vi "Check_Execution_Row.vi"(0 "Execution Row":T1 {"Row Duration (mins)" format="%#.1f"; "Row No" min=0; "Trace Gas Concentration (%)" min=0.0 format="%#.2f"; "Emission Rate (l/min)" format="%#.2f"; "Tunnel Speed" format="%#.2f"; "Start X" format="%#.2f"; "Start Y" format="%#.2f"; "Start Z" format="%#.2f"; "End X" format="%#.2f"; "End Y" format="%#.2f"; "End Z" format="%#.2f"; "Averaging time (min)" min=0.0 format="%#.2f"}, 3 "Synchronization Start No":i32=1 min=1 max=100, 4 "Row Index":i32, 5 "Max Tunnel Speed":dbl format="%.2f") -> (6 "Editted Row":bool, 7 "Execution Row Out":T1 {"Row Duration (mins)" format="%#.1f"; "Row No" min=0; "Trace Gas Concentration (%)" min=0.0 format="%#.2f"; "Emission Rate (l/min)" format="%#.2f"; "Tunnel Speed" format="%#.2f"; "Start X" format="%#.2f"; "Start Y" format="%#.2f"; "Start Z" format="%#.2f"; "End X" format="%#.2f"; "End Y" format="%#.2f"; "End Z" format="%#.2f"; "Averaging time (min)" min=0.0 format="%#.2f"}, 9 "Continue?":bool, 10 "Error Comments":string)   [LabVIEW 2013]
uses:
  Traverse_cluster.ctl
  Spacing.ctl
  Controls/Multi_run_mode.ctl
  Controls/User_Specific_mode.ctl
  Controls/Tunnel_Coordinates.ctl
  ADAM Client/Sub VIs/ADAM Controls/Channel_names.ctl
  Globals/Extra_Commands_Global.vi
  Globals/Constants_global.vi
  Globals/Trav_pos_global.vi
panel:
  out "Traverse line Out":T1 {"Row Duration (mins)" format="%#.1f"; "Row No" min=0; "Trace Gas Concentration (%)" min=0.0 format="%#.2f"; "Emission Rate (l/min)" format="%#.2f"; "Tunnel Speed" format="%#.2f"; "Start X" format="%#.2f"; "Start Y" format="%#.2f"; "Start Z" format="%#.2f"; "End X" format="%#.2f"; "End Y" format="%#.2f"; "End Z" format="%#.2f"; "Averaging time (min)" min=0.0 format="%#.2f"}
  out "Fixed Axis":bool[](array[boolean])
  out "Filenames":string[](array[string])
  out "Current Sync Number":i32
  out "Checks":string[](array[string])
  in  "Edit in Excel":bool
  in  "OK":bool
  # "X           Y            Z"
  # "Start"
  # "End"
  # "X           Y            Z"
  # "Start"
  # "End"
  # "X           Y            Z"
  # "Start"
  # "End"
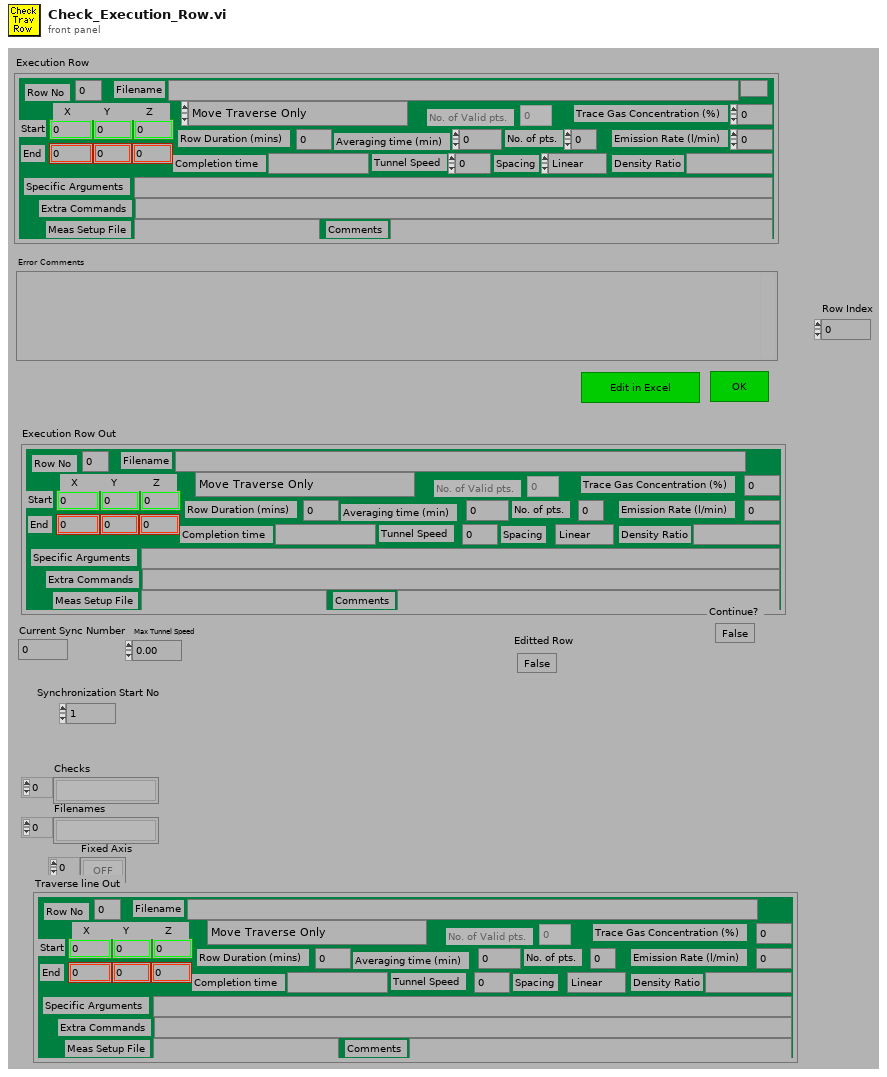
[diagram p1: front panel]
types:
  T1 = typedef "Traverse_cluster.ctl" = cluster{"Start X":dbl, "Start Y":dbl, "Start Z":dbl, "End X":dbl, "End Y":dbl, "End Z":dbl, "No. of pts.":i32, "Spacing":T2, "Filename":path, "Tunnel Speed":dbl, "Averaging time (min)":dbl, "Extra Commands":string, "Specific Arguments":string, "Emission Rate (l/min)":dbl, "Trace Gas Concentration (%)":dbl, "Density Ratio":string, "Comments":string, "Row No":i32, "Row Type Selector":T3, "Completion time":string, "Row Duration (mins)":dbl, "No. of Valid pts.":i32, "Meas Setup File":string}
  T2 = typedef "Spacing.ctl" = enum16{"Linear", "Log", "Gauss", "Specified", "N/A"}
  T3 = typedef "Multi_run_mode.ctl" = enum16{"Move Traverse Only", "Set Tunnel Speed Only", "Set Source Only", "Set Measurement Conditions", "Single Measurement", "Vertical Profile", "Lateral Profile", "Longitudinal Profile", "Explore Volume", "Multi-Axis Profile", "Auto Calibrate", "Meas Fast FID Bkgnd", "Check Beam Power", "Scanning Valve Measurement", "Run VI Named:", "Set ADAM Ch", "Wait (minutes)", "Send Message", "Synchronize With:", "Fall Back to this Row", "Turn Off Row Repeating", "Blank Row", "Traverse 3D Volume"}
  T4 = enum16{"All Channel Names", "Valid Channel Names"}
  T5 = typedef "User_Specific_mode.ctl" = enum16{"Check VI only", "Run VI"}
  T6 = typedef "Tunnel_Coordinates.ctl" = enum16{"Work in Tunnel Coordinates", "Work in Model Coordinates"}
  T7 = enum16{"Zero or one", "One", "Zero or more", "One or more"}
  T8 = typedef "Channel_names.ctl" = enum16{"Active Only", "Active + Off", "All Channels"}
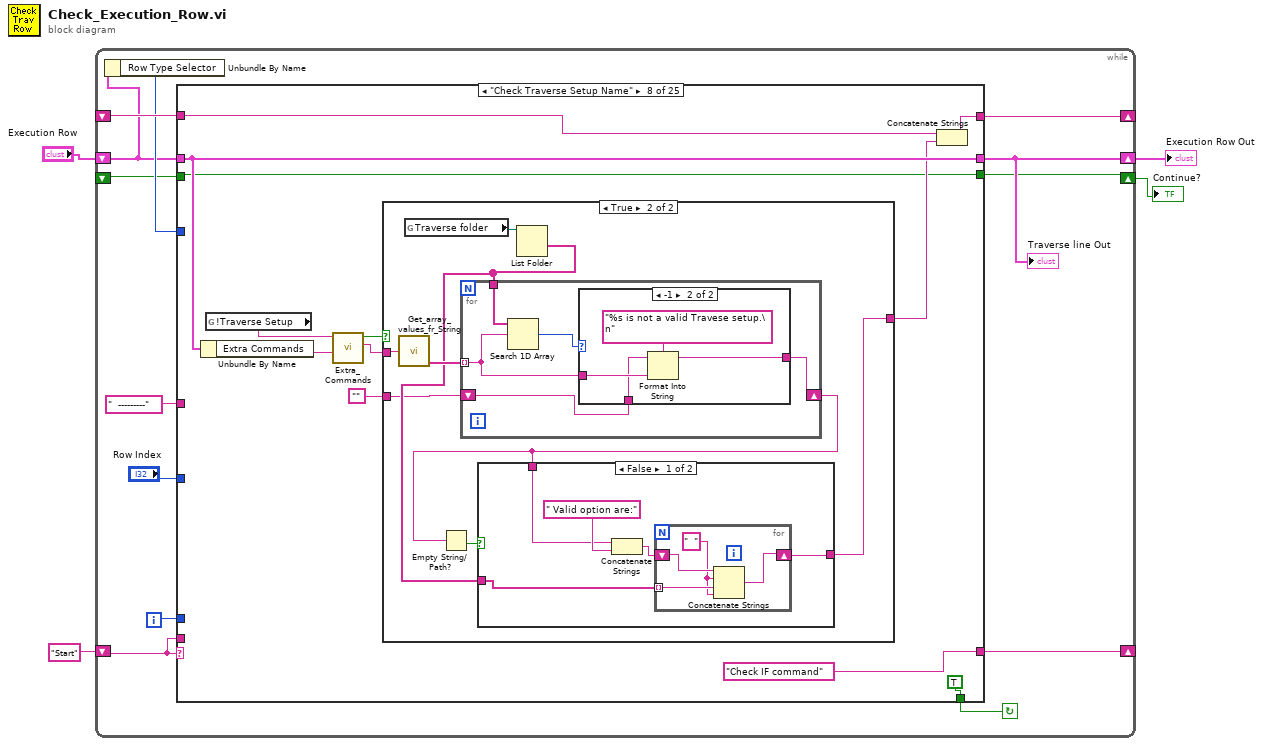
[diagram p0: block diagram]
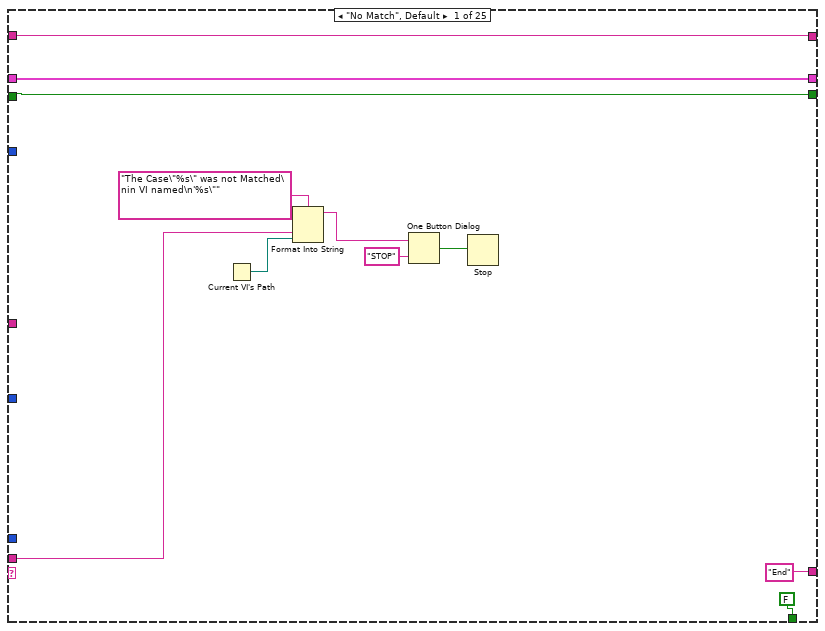
[diagram p2: hidden frame]
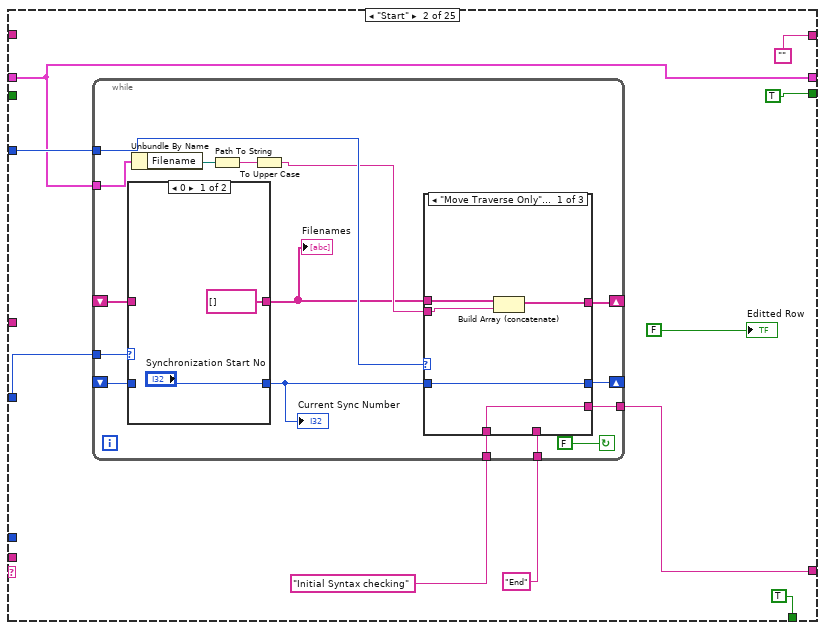
[diagram p3: hidden frame]
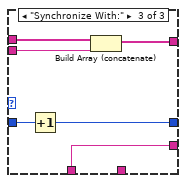
[diagram p6: hidden frame]
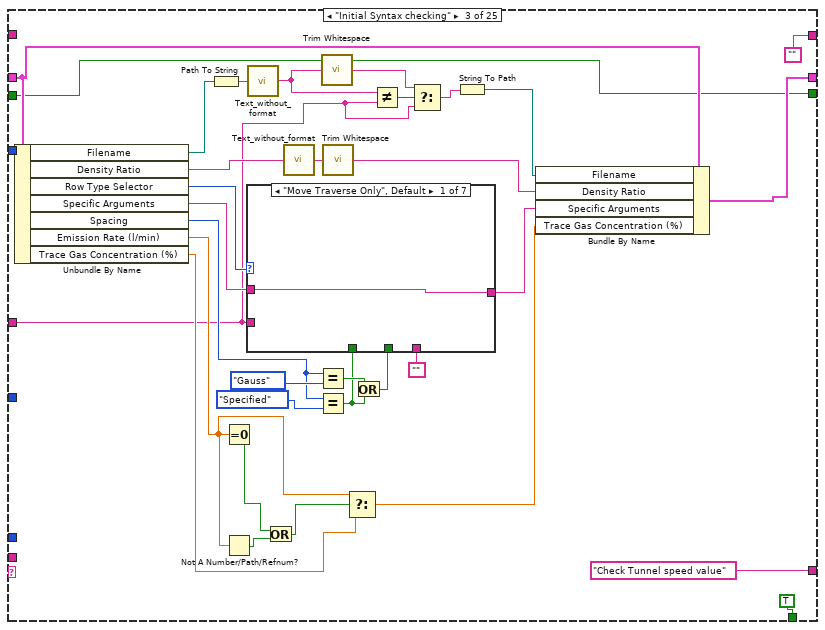
[diagram p7: hidden frame]
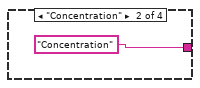
[diagram p9: hidden frame]
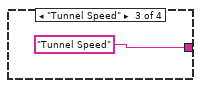
[diagram p10: hidden frame]
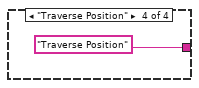
[diagram p11: hidden frame]
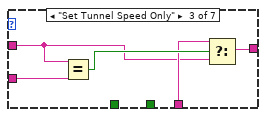
[diagram p12: hidden frame]
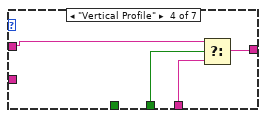
[diagram p13: hidden frame]
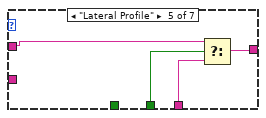
[diagram p14: hidden frame]
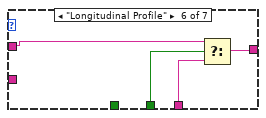
[diagram p15: hidden frame]
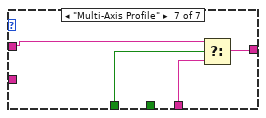
[diagram p16: hidden frame]
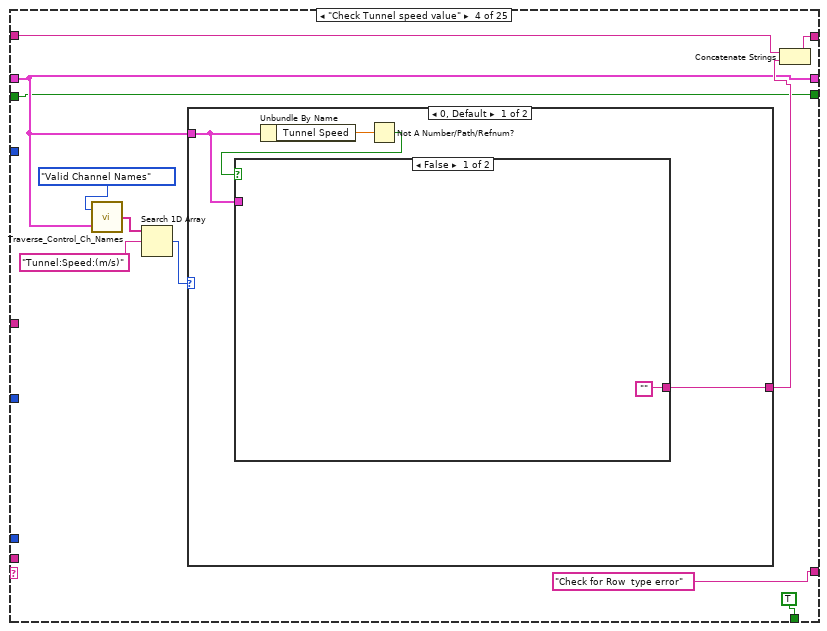
[diagram p17: hidden frame]
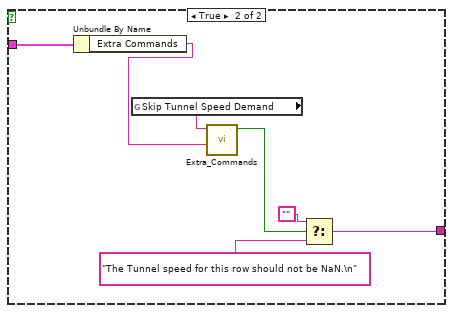
[diagram p18: hidden frame]
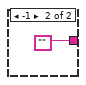
[diagram p19: hidden frame]
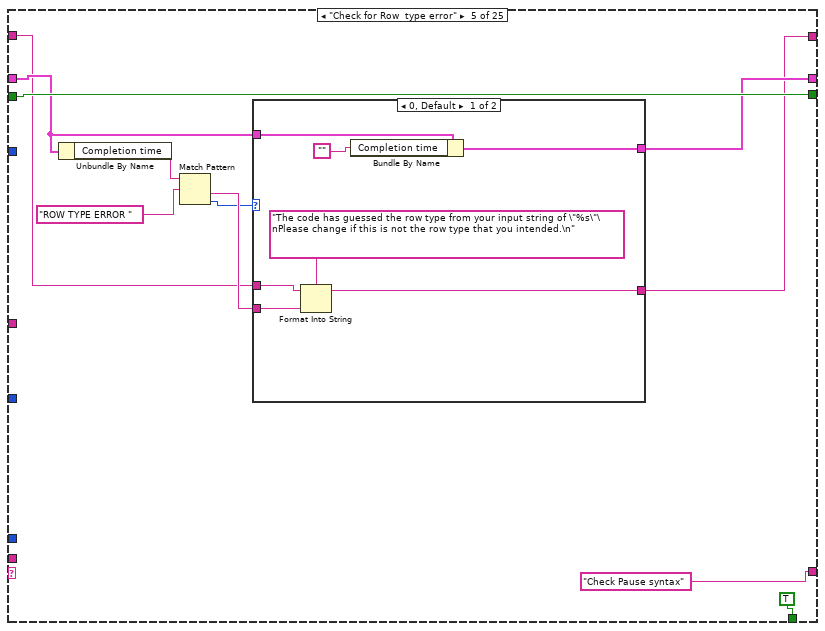
[diagram p20: hidden frame]
diagram:
  n1 = while {
    shift-left: _ -> [w16]
    shift-right: [w17] -> _
    shift-left: "Start" -> [w9]
    shift-right: [w14] -> _
    shift-right: [w8] -> w2
    shift-left: "Execution Row" -> [w5]
    shift-right: [w7] -> w1
    shift-left: _ -> [w6]
    i -> [w10]
    stop <- w15 continue-if-true
    n2 = Unbundle By Name(w5) -> ("Row Type Selector"=w12:T3)
    n3 = case shown="\"Check Traverse Setup Name\"" w9 {
      tunnel: w5 -> [w22 w32 w100 w137 w161 w193 w211 w252 w293 w349 w382 w390 w429 w774 w874 w911 w939 w1024 w1056 w1066 w1135 _ w1174 w1181 w1191]
      tunnel: "  ---------" ("f") -> [_ _ w74 _ _ w197 _ _ _ _ _ _ _ _ _ _ _ _ _ _ _ _ _ _ _]
      tunnel: "Row Index" -> [_ w36 _ _ _ _ w208 _ _ _ _ _ w423 _ _ _ _ _ _ _ _ _ w1175 _ w1190]
      tunnel: [w21 "" "" w138 w158 w186 w219 w257 w298 w351 w386 w395 w433 w779 w884 w917 w962 w1022 w1060 w1067 w1141 w1152 w1176 w1186 w1193] -> w17
      tunnel: w12 -> [_ w35 _ _ _ w179 _ _ _ _ _ w393 w432 w775 w872 _ _ _ _ w1071 _ _ _ _ _]
      tunnel: w16 -> [w21 _ _ w139 w159 w188 w220 w258 w299 w351 w385 w396 w434 w779 w885 w918 w963 w1022 w1061 w1072 w1141 w1152 w1176 w1186 w1193]
      tunnel: [FALSE TRUE TRUE TRUE TRUE TRUE TRUE TRUE TRUE TRUE TRUE TRUE TRUE TRUE TRUE TRUE TRUE TRUE TRUE w1063 TRUE TRUE TRUE TRUE FALSE] -> w15
      tunnel: ["End" w33 "Check Tunnel speed value" ("f") "Check for Row  type error" ("f") "Check Pause syntax" ("f") w191 "Check Traverse Setup Name" ("f") "Check IF command" ("f") "Check Measurement Setup?" ("f") w353 "Check Maximum tunnel speed" ("f") "Row type specific check" ("f") w430 "Check for position NaNs" ("f") w875 "Check source details" ("t") "Check source details" ("f") w1019 "check entered filename etc" ("f") w1069 "What to do next?" ("f") w1150 "Initial Syntax checking" "End" "End"] -> w14
      tunnel: w10 -> [_ _ _ _ _ _ _ _ _ _ _ _ _ _ _ _ _ _ _ _ _ _ _ _ _]
      tunnel: w9 -> [w23 _ _ _ _ _ _ _ _ _ _ _ _ _ _ _ _ _ _ _ _ _ _ _ _]
      tunnel: [w22 w32 w77 w137 w162 w181 w210 w252 w293 w349 w381 w390 w424 w773 w874 w911 w938 w1023 w1056 w1065 w1135 w1143 w1177 w1181 w1189] -> w8
      tunnel: [w18 TRUE w75 w136 w168 w182 w212 w250 w290 w355 w383 w388 w426 w771 w873 w910 w936 w1027 w1054 w1063 w1134 w1142 w1171 w1180 w1187] -> w7
      tunnel: w6 -> [w18 _ w75 w136 w168 w182 w212 w250 w290 w355 w383 w388 w426 w771 w873 w910 w936 w1027 w1054 _ w1134 _ w1171 w1180 w1187]
      frame "No Match", Default {
        n4 = Current VI's Path() -> (path=w24:path)
        n5 = Format Into String(format string="The Case\"%s\" was not Matched\nin VI named\n'%s\"" ("Format String"), w23, w24) -> (resulting string=w27:string)  [unwired: 2 in, 1 out]
        n6 = One Button Dialog(message=w27, button name ("OK")="STOP") -> (true=w25:bool)
        n7 = Stop(stop? (T)=w25) -> ()
      }
      frame "Start" {
        n8 = while {
          tunnel: "End" -> [w40]
          tunnel: "Initial Syntax checking" -> [w41]
          tunnel: [w42] -> w33
          tunnel: w32 -> [w49]
          shift-left: _ -> [w48]
          shift-right: [w47] -> _
          tunnel: w35 -> [w53]
          shift-left: _ -> [w52]
          shift-right: [w51] -> _
          tunnel: w36 -> [w54]
          stop <- FALSE continue-if-true
          n9 = case shown="0" w54 {
            tunnel: ["Synchronization Start No" w58] -> w50
            tunnel: w52 -> [_ w58]
            tunnel: w48 -> [_ w57]
            tunnel: [string[] [] w57] -> w43
            frame 0 {
            }
            frame 1, Default {
            }
          }
          "Current Sync Number" <- w50
          "Filenames" <- w43
          n10 = Unbundle By Name(w49) -> ("Filename"=w46:path)
          n11 = Path To String(path=w46) -> (string=w45:string)
          n12 = To Upper Case(1:w45) -> (0:w44:string)
          n13 = case shown="\"Move Traverse Only\", Default" w53 {
            tunnel: w50 -> [w63 w66 w72]
            tunnel: [w63 w66 w71] -> w51
            tunnel: w44 -> [w61 _ w70]
            tunnel: w43 -> [w62 w65 w69]
            tunnel: [w60 w65 w68] -> w47
            tunnel: [w59 w64 w67] -> w42
            tunnel: w41 -> [w59 _ w67]
            tunnel: w40 -> [_ w64 _]
            frame "Move Traverse Only", Default {
              n14 = Build Array (concatenate)(w62, w61) -> (w60:string[])
            }
            frame "Blank Row" {
            }
            frame "Synchronize With:" {
              n15 = Increment(x=w72) -> (x+1=w71:i32)
              n16 = Build Array (concatenate)(w69, w70) -> (w68:string[])
            }
          }
        }
        "Editted Row" <- FALSE ("Editted Row")
      }
      frame "Initial Syntax checking" {
        n17 = Unbundle By Name(w100) -> ("Filename"=w73:path, "Density Ratio"=w79:string, "Row Type Selector"=w97:T3, "Specific Arguments"=w95:string, "Spacing"=w87:T2, "Emission Rate (l/min)"=w83:dbl, "Trace Gas Concentration (%)"=w93:dbl)
        n18 = Path To String(path=w73) -> (string=w81:string)
        n19 = Equal To 0?(x=w83) -> (x = 0?=w85:bool)
        n20 = Not A Number/Path/Refnum?(number/path/refnum=w83) -> (NaN/Path/Refnum?=w84:bool)
        n21 = call "Text_without_format.vi"("Input string"=w81) -> ("Output string"=w104:string)
        n22 = Or(x=w85, y=w84) -> (x .or. y?=w82:bool)
        n23 = call "Text_without_format.vi"("Input string"=w79) -> ("Output string"=w99:string)
        n24 = Equal?(x=w87, y=Spacing."Gauss" ("Spacing")) -> (x = y?=w89:bool)
        n25 = Equal?(x=w87, y=Spacing."Specified" ("Spacing")) -> (x = y?=w86:bool)
        n26 = call <vilib>:"Trim Whitespace.vi"("string"=w104) -> ("trimmed string"=w103:string)  [unwired: 1 in]
        n27 = call <vilib>:"Trim Whitespace.vi"("string"=w99) -> ("trimmed string"=w78:string)  [unwired: 1 in]
        n28 = Select(t=w83, s=w82, f=w93) -> (s? t:f=w92:dbl)
        n29 = Or(x=w89, y=w86) -> (x .or. y?=w88:bool)
        n30 = case shown="\"Move Traverse Only\", Default" w97 {
          tunnel: [w106 w108 w113 w119 w123 w127 w131] -> w96
          tunnel: w95 -> [w106 w107 w114 w121 w125 w129 w133]
          tunnel: "" -> [_ _ w115 w120 w124 w128 w132]
          tunnel: w88 -> [_ _ _ w118 w122 w126 _]
          tunnel: w86 -> [_ _ _ _ _ _ w130]
          tunnel: w74 -> [_ _ w117 _ _ _ _]
          frame "Move Traverse Only", Default {
          }
          frame "Auto Calibrate" {
            n31 = case shown="\"No Match\", Default" w107 {
              tunnel: [w109 "Concentration" "Tunnel Speed" "Traverse Position"] -> w108
              tunnel: w107 -> [w109 _ _ _]
              frame "No Match", Default {
              }
              frame "Concentration" {
              }
              frame "Tunnel Speed" {
              }
              frame "Traverse Position" {
              }
            }
          }
          frame "Set Tunnel Speed Only" {
            n32 = Equal?(x=w114, y=w117) -> (x = y?=w116:bool)
            n33 = Select(t=w115, s=w116, f=w114) -> (s? t:f=w113:string)
          }
          frame "Vertical Profile" {
            n34 = Select(t=w121, s=w118, f=w120) -> (s? t:f=w119:string)
          }
          frame "Lateral Profile" {
            n35 = Select(t=w125, s=w122, f=w124) -> (s? t:f=w123:string)
          }
          frame "Longitudinal Profile" {
            n36 = Select(t=w129, s=w126, f=w128) -> (s? t:f=w127:string)
          }
          frame "Multi-Axis Profile" {
            n37 = Select(t=w133, s=w130, f=w132) -> (s? t:f=w131:string)
          }
        }
        n38 = Not Equal?(x=w104, y=w74) -> (x != y?=w105:bool)
        n39 = Select(t=w103, s=w105, f=w74) -> (s? t:f=w102:string)
        n40 = String To Path(string=w102) -> (path=w80:path)
        n41 = Bundle By Name(cluster=w100, "Filename"=w80, "Density Ratio"=w78, "Specific Arguments"=w96, "Trace Gas Concentration (%)"=w92) -> (w77:T1)
      }
      frame "Check Tunnel speed value" {
        n42 = call "Traverse_Control_Ch_Names.vi"("Traverse line"=w137, "Mode"=T4."Valid Channel Names") -> ("Channel names"=w143:string[])
        n43 = Search 1D Array(1D array=w143, element="Tunnel:Speed:(m/s)" ("Label for value")) -> (index of element=w141:i32)  [unwired: 1 out]
        n44 = case shown="0, Default" w141 {
          tunnel: w137 -> [w146 _]
          tunnel: [w145 ""] -> w140
          frame 0, Default {
            n45 = Unbundle By Name(w146) -> ("Tunnel Speed"=w148:dbl)
            n46 = Not A Number/Path/Refnum?(number/path/refnum=w148) -> (NaN/Path/Refnum?=w147:bool)
            n47 = case shown="False" w147 {
              tunnel: w146 -> [_ w156]
              tunnel: ["" w150] -> w145
              frame False {
              }
              frame True {
                n48 = Unbundle By Name(w156) -> ("Extra Commands"=w154:string)
                n49 = global read "Extra_Commands_Global.vi" "Skip Tunnel Speed Demand"() -> (w155:string)
                n50 = call "Extra_Commands.vi"("String to Search"=w154, "Command"=w155) -> ("Command Found"=w153:bool)  [unwired: 1 in, 4 out]
                n51 = Select(t="", s=w153, f="The Tunnel speed for this row should not be NaN.\n") -> (s? t:f=w150:string)
              }
            }
          }
          frame -1 {
          }
        }
        n52 = Concatenate Strings(w139, w140) -> (w138:string)
      }
      frame "Check for Row  type error" {
        n53 = Unbundle By Name(w161) -> ("Completion time"=w164:string)
        n54 = Match Pattern(string=w164, regular expression="ROW TYPE ERROR " ("format string")) -> (after substring=w163:string, offset past match=w160:i32)  [unwired: 3 out]
        n55 = case shown="0, Default" w160 {
          tunnel: w163 -> [w175 _]
          tunnel: [w173 w177] -> w162
          tunnel: w161 -> [w172 w177]
          tunnel: [w170 w176] -> w158
          tunnel: w159 -> [w169 w176]
          frame 0, Default {
            n56 = Format Into String(format string="The code has guessed the row type from your input string of \"%s\"\nPlease change if this is not the row type that you intended.\n", initial string=w169, w175) -> (resulting string=w170:string)  [unwired: 1 in, 1 out]
            n57 = Bundle By Name(cluster=w172, "Completion time"="") -> (w173:T1)
          }
          frame -1 {
          }
        }
      }
      frame "Check Pause syntax" {
        n58 = Unbundle By Name(w193) -> ("Extra Commands"=w198:string)
        n59 = Equal?(x=Multi_run_mode."Set ADAM Ch" ("Row Type Selector"), y=w179) -> (x = y?=w178:bool)
        n60 = Not Equal?(x=w198, y=w197) -> (x != y?=w199:bool)
        n61 = Select(t=w198, s=w199, f="") -> (s? t:f=w195:string)
        n62 = call <vilib>:"Trim Whitespace.vi"("string"=w195) -> ("trimmed string"=w190:string)  [unwired: 1 in]
        n63 = case shown="True" w178 {
          tunnel: [w201 TRUE] -> w192
          tunnel: w190 -> [w200 _]
          frame False {
            n64 = Equal?(x=w200, y="") -> (x = y?=w201:bool)
          }
          frame True {
          }
        }
        n65 = call "Pause_for_server_ch_val.vi"("Extra command string"=w190, "Simulate/Run"=User_Specific_mode."Check VI only") -> ("Extra command string Out"=w189:string, "Error Comments"=w187:string)
        n66 = Bundle By Name(cluster=w193, "Extra Commands"=w189) -> (w181:T1)
        n67 = Concatenate Strings(w188, w187) -> (w186:string)
        n68 = Select(t="Check Measurement Setup?", s=w192, f="Check Extra Commands") -> (s? t:f=w191:string)
      }
      frame "Check Extra Commands" {
        n69 = Unbundle By Name(w211) -> ("Extra Commands"=w213:string)
        n70 = for {
          N: 3 -> [_]
          tunnel: w213 -> [w228]
          shift-right: [w224] -> w216
          shift-left: "" -> [w225]
          i -> [w230]
          n71 = case shown="0, Default" w230 {
            tunnel: [w233 w235 w237] -> w227
            tunnel: ["The Extra Command \"%s\" should have a numeric argument of (Centre; Intensity) eg 0 ; 0.85 for Gaussian spacing or (Offset) eg 300 for Log \n" ("Format String") "The Extra Command \"%s\" should have a numeric argument.\n" ("Format String") "The Extra Command \"%s\" should have a numeric argument.\n" ("Format String")] -> w222
            frame 0, Default {
              n72 = global read "Extra_Commands_Global.vi" "Point Spacing Parameters"() -> (w233:string)
            }
            frame 1 {
              n73 = global read "Extra_Commands_Global.vi" "Establish Exp Conditions (s)"() -> (w235:string)
            }
            frame 2 {
              n74 = global read "Extra_Commands_Global.vi" "Minutes Before Repeating Row"() -> (w237:string)
            }
          }
          n75 = call "Extra_Commands.vi"("String to Search"=w228, "Command"=w227) -> ("String Value"=w229:string, "Command Found"=w231:bool)  [unwired: 1 in, 3 out]
          n76 = case shown="True" w231 {
            tunnel: w229 -> [_ w246]
            tunnel: w227 -> [_ w244]
            tunnel: [w238 w241] -> w226
            tunnel: "" -> [w238 w240]
            tunnel: w222 -> [_ w239]
            frame False {
            }
            frame True {
              n77 = Decimal String To Number(string=w246) -> (offset past number=w245:i32)  [unwired: 3 out]
              n78 = Equal To 0?(x=w245) -> (x = 0?=w243:bool)
              n79 = Format Into String(format string=w239, w244) -> (resulting string=w242:string)  [unwired: 2 in, 1 out]
              n80 = Select(t=w242, s=w243, f=w240) -> (s? t:f=w241:string)
            }
          }
          n81 = Concatenate Strings(w226, w225) -> (w224:string)
        }
        n82 = call "Trav_Prog_Extra_Commands.vi"() -> ("Extra Commands Array"=w214:string[])  [unwired: 2 out]
        n83 = call "Valid_Extra_Command.vi"("Extra Commands string"=w213, "Valid Commands Array"=w214) -> ("Output String"=w218:string, "Extra Commands string Out"=w209:string)  [unwired: 3 out]
        n84 = Bundle By Name(cluster=w211, "Extra Commands"=w209) -> (w210:T1)
        n85 = call "Skip_If Sd_Error_Below.vi"("String to Search"=w209, "Simulate/Run"=User_Specific_mode."Check VI only", "Measurement setup Applied?"=FALSE, "Row Number"=w208) -> ("Error String"=w205:string)  [unwired: 1 in, 4 out]
        n86 = Concatenate Strings(w220, w218, w216, w205) -> (w219:string)
      }
      frame "Check Traverse Setup Name" {
        n87 = Unbundle By Name(w252) -> ("Extra Commands"=w249:string)
        n88 = global read "Extra_Commands_Global.vi" "!Traverse Setup"() -> (w255:string)
        n89 = call "Extra_Commands.vi"("String to Search"=w249, "Command"=w255) -> ("String Value"=w253:string, "Command Found"=w254:bool)  [unwired: 1 in, 3 out]
        n90 = case shown="True" w254 {
          tunnel: w253 -> [_ w266]
          tunnel: [w259 w261] -> w251
          tunnel: "" -> [w259 w260]
          frame False {
          }
          frame True {
            n91 = call "Get_array_values_fr_String.vi"("String Value"=w266) -> ("String array"=w265:string[])  [unwired: 1 out]
            n92 = global read "Constants_global.vi" "Traverse folder"() -> (w267:path)
            n93 = List Folder(path=w267) -> (folder names=w263:string[])  [unwired: 1 in, 5 out]
            n94 = for {
              tunnel: w265 -> [w280] mode=indexing
              tunnel: w263 -> [w282]
              shift-right: [w278] -> w264
              shift-left: w260 -> [w279]
              n95 = Search 1D Array(1D array=w282, element=w280) -> (index of element=w281:i32)  [unwired: 1 out]
              n96 = case shown="-1" w281 {
                tunnel: w280 -> [_ w286]
                tunnel: [w283 w285] -> w278
                tunnel: w279 -> [w283 w284]
                frame Default {
                }
                frame -1 {
                  n97 = Format Into String(format string="%s is not a valid Travese setup.\n", initial string=w284, w286) -> (resulting string=w285:string)  [unwired: 1 in, 1 out]
                }
              }
            }
            n98 = Empty String/Path?(string/path=w264) -> (empty?=w262:bool)
            n99 = case shown="False" w262 {
              tunnel: w263 -> [w272 _]
              tunnel: [w271 w277] -> w261
              tunnel: w264 -> [w269 w277]
              frame False {
                n100 = Concatenate Strings(w269, " Valid option are:" ("format string")) -> (w268:string)
                n101 = for {
                  shift-right: [w274] -> w271
                  shift-left: w268 -> [w275]
                  tunnel: w272 -> [w276] mode=indexing
                  w273 = "  " ("Substring")
                  n102 = Concatenate Strings(w275, w273, w276, w273) -> (w274:string)
                }
              }
              frame True {
              }
            }
          }
        }
        n103 = Concatenate Strings(w258, w251) -> (w257:string)
      }
      frame "Check IF command" {
        n104 = Unbundle By Name(w293) -> ("Extra Commands"=w289:string)
        n105 = global read "Extra_Commands_Global.vi" "If Command"() -> (w296:string)
        n106 = call "Extra_Commands.vi"("String to Search"=w289, "Command"=w296) -> ("String Value"=w294:string, "Command Found"=w295:bool)  [unwired: 1 in, 3 out]
        n107 = case shown="True" w295 {
          tunnel: w294 -> [_ w305]
          tunnel: [w300 w304] -> w291
          tunnel: "" -> [w300 w302]
          frame False {
          }
          frame True {
            n108 = call "Get_array_values_fr_String.vi"("String Value"=w305) -> ("Numeric Array"=w301:dbl[], "String array"=w303:string[])
            n109 = Index Array(array=w303, index=0 ("Index")) -> (element=w306:string)
            n110 = case shown="\"Global Value Between\"" w306 {
              tunnel: w305 -> [w311 _ _ _]
              tunnel: [w310 w336 w337 "The !If  command has not been recognised.\nExtra command Example:\n!IF = Time Between;10:45;and;14:00;Execute Row (or) Skip Row\n\n!IF = ADAM Channel Between;Channel Name; 0.5;1.0\n\n!IF = Global Value Between; 0.5;1.0" ("Error Comments")] -> w304
              tunnel: w303 -> [_ w327 w345 _]
              tunnel: w302 -> [_ w320 w338 _]
              tunnel: w301 -> [_ _ _ _]
              frame "Time Between" {
                n111 = Get Date/Time In Seconds() -> (seconds since 1Jan1904=w308:timestamp)
                n112 = To Double Precision Float(number=w308) -> (double precision float=w309:dbl)
                n113 = call "If_Time_arguments.vi"("seconds since 1Jan1904"=w309, "String Value"=w311) -> ("Error Comments"=w310:string)  [unwired: 2 out]
              }
              frame "ADAM Channel Between" {
                n114 = Index Array(array=w327, index=1 ("Index")) -> (element=w330:string)
                n115 = Index Array(array=w327, index=2 ("Index")) -> (element=w326:string)
                n116 = Index Array(array=w327, index=3 ("Index")) -> (element=w325:string)
                n117 = Build Array(w330) -> (w332:string[])
                n118 = Decimal Digit?(1:w326) -> (0:w323:bool)
                n119 = Decimal Digit?(1:w325) -> (0:w324:bool)
                n120 = call "Get_Current_Scan_client.vi"("ADAM Ch Names"=w332) -> ("Numerical Values"=w334:dbl[])  [unwired: 3 out]
                n121 = And(x=w323, y=w324) -> (x .and. y?=w322:bool)
                n122 = Index Array(array=w334, index=0 ("Index")) -> (element=w335:dbl)
                n123 = Select(t=w320, s=w322, f="you must give two limits\n") -> (s? t:f=w316:string)
                n124 = Not A Number/Path/Refnum?(number/path/refnum=w335) -> (NaN/Path/Refnum?=w319:bool)
                n125 = Select(t="Invalid ADAM Channel Name\n", s=w319, f=w320) -> (s? t:f=w317:string)
                n126 = Concatenate Strings(w317, w316) -> (w314:string)
                n127 = Concatenate Strings(w314, "Extra command Example:\n!IF = ADAM Channel Between;Channel Name; 0.5;1.0") -> (w313:string)
                n128 = Empty String/Path?(string/path=w314) -> (empty?=w315:bool)
                n129 = Select(t=w320, s=w315, f=w313) -> (s? t:f=w336:string)
              }
              frame "Global Value Between" {
                n130 = Index Array(array=w345, index=1 ("Index")) -> (element=w344:string)
                n131 = Index Array(array=w345, index=2 ("Index")) -> (element=w343:string)
                n132 = Decimal Digit?(1:w344) -> (0:w341:bool)
                n133 = Decimal Digit?(1:w343) -> (0:w342:bool)
                n134 = And(x=w341, y=w342) -> (x .and. y?=w340:bool)
                n135 = Select(t=w338, s=w340, f="The Extra command IF statement must have two numerical values for the limits\n\nExtra command Example:\n!IF = Global Value Between; 0.5;1.0") -> (s? t:f=w337:string)
              }
              frame "No Match", Default {
              }
            }
          }
        }
        n136 = Concatenate Strings(w299, w291) -> (w298:string)
      }
      frame "Check Measurement Setup?" {
        n137 = Unbundle By Name(w349) -> ("Row Type Selector"=w354:T3, "Specific Arguments"=w352:string)
        n138 = case shown="\"Traverse 3D Volume\"" w354 {
          tunnel: ["Check Measurement Setup" ("t") "Check Measurement Setup" ("t") "Check Measurement Setup" ("t") "Check Measurement Setup" ("t") "Check Measurement Setup" ("t") "Check Measurement Setup" ("t") "Check Measurement Setup" ("t") "Check Measurement Setup" ("t") "Check Measurement Setup" ("t") "Check Measurement Setup" ("t") "Check Measurement Setup" ("t") w368 w377] -> w353
          tunnel: w352 -> [_ _ _ _ _ _ _ _ _ _ _ w375 _]
          tunnel: "Check Maximum tunnel speed" ("f") -> [_ _ _ _ _ _ _ _ _ _ _ w369 w377]
          tunnel: w349 -> [_ _ _ _ _ _ _ _ _ _ _ w372 _]
          frame "Lateral Profile" {
          }
          frame "Traverse 3D Volume" {
          }
          frame "Longitudinal Profile" {
          }
          frame "Explore Volume" {
          }
          frame "Multi-Axis Profile" {
          }
          frame "Vertical Profile" {
          }
          frame "Single Measurement" {
          }
          frame "Scanning Valve Measurement" {
          }
          frame "Auto Calibrate" {
          }
          frame "Meas Fast FID Bkgnd" {
          }
          frame "Check Beam Power" {
          }
          frame "Run VI Named:" {
            n139 = Match Pattern(string=w375, regular expression=";") -> (before substring=w374:string)  [unwired: 4 out]
            n140 = call <vilib>:"Trim Whitespace.vi"("string"=w374) -> ("trimmed string"=w373:string)  [unwired: 1 in]
            n141 = call "Run_VI_Named_specific.vi"("Run VI Named String"=w373, "Multi Run Row"=w372) -> ("Check Meas Setup?"=w371:bool)  [unwired: 9 out]
            n142 = Select(t="Check Measurement Setup", s=w371, f=w369) -> (s? t:f=w368:string)
          }
          frame "Set Tunnel Speed Only", Default {
          }
        }
      }
      frame "Check Measurement Setup" {
        n143 = Unbundle By Name(w382) -> ("Meas Setup File"=w380:string)
        n144 = call "Check_Measurement_Setups.vi"("Measurement Setup String"=w380) -> ("Measurement Setup String Out"=w379:string, "Error Comments"=w378:string)
        n145 = Bundle By Name(cluster=w382, "Meas Setup File"=w379) -> (w381:T1)
        n146 = Concatenate Strings(w385, w378) -> (w386:string)
      }
      frame "Check Maximum tunnel speed" {
        n147 = case shown="\"Set Tunnel Speed Only\", Default" w393 {
          tunnel: w390 -> [w415 _]
          tunnel: [w406 FALSE] -> w392
          tunnel: [w405 0.0] -> w391
          frame "Auto Calibrate" {
            n148 = Unbundle By Name(w415) -> ("Specific Arguments"=w414:string)
            n149 = call "Get_array_values_fr_String.vi"("String Value"=w414) -> ("Numeric Array"=w408:dbl[], "String array"=w413:string[])
            n150 = Index Array(array=w413, index=0 ("Index")) -> (element=w411:string)
            n151 = Equal?(x=w411, y="Tunnel Speed" ("Output Array")) -> (x = y?=w406:bool)
            n152 = Array Subset(array=w408, index=1 ("Array Index")) -> (w407:dbl[])  [unwired: 1 in]
            n153 = Array Max & Min(array=w407) -> (max value=w405:dbl)  [unwired: 3 out]
          }
          frame "Set Tunnel Speed Only", Default {
          }
        }
        n154 = case shown="False" w392 {
          tunnel: [w403 w404] -> w400
          tunnel: w390 -> [w402 _]
          tunnel: w391 -> [_ w404]
          frame False {
            n155 = Unbundle By Name(w402) -> ("Tunnel Speed"=w403:dbl)
          }
          frame True {
          }
        }
        n156 = Greater?(x=w400, y="Max Tunnel Speed") -> (0:w398:bool)
        n157 = Not A Number/Path/Refnum?(number/path/refnum=w400) -> (NaN/Path/Refnum?=w399:bool)
        n158 = Compound Arithmetic op=AND(invert w399, w398) -> (w397:bool)
        n159 = case shown="False" w397 {
          tunnel: w396 -> [w418 w420]
          tunnel: [w418 w419] -> w395
          tunnel: "Max Tunnel Speed" -> [_ w422]
          frame False {
          }
          frame True {
            n160 = Format Into String(format string="The maximum allowable tunnel speed is %.2f m/s.\n" ("Format String"), initial string=w420, w422) -> (resulting string=w419:string)  [unwired: 1 in, 1 out]
          }
        }
      }
      frame "Row type specific check" {
        n161 = case shown="\"Set ADAM Ch\"" w432 {
          tunnel: w429 -> [w443 w452 w456 w460 w465 w470 w477 w484 w495 w503 w517 w521 w598 w605 w626 w653 w701 w729 w734 w738 w750 w754 w760]
          tunnel: [string[] [] string[] [] string[] [] string[] [] w466 w473 w480 w487 w500 w508 w518 w543 w600 string[] [] w643 string[] [] w696 string[] [] string[] [] string[] [] string[] [] string[] [] string[] []] -> w431
          tunnel: [w437 "" "" "" "" "" "" "" w496 w505 "" w557 w594 w604 w638 w647 w712 w731 "" w740 "" "" w762] -> w435
          tunnel: [w446 w453 w457 w461 w464 w471 w478 w485 w494 w504 w516 w542 w588 w603 w637 w656 w697 "check entered filename etc" "check entered filename etc" "check entered filename etc" "check entered filename etc" "check entered filename etc" "check entered filename etc"] -> w430
          tunnel: "Check source details" -> [_ w453 w457 _ _ _ _ _ _ _ w516 _ w588 w603 w637 w655 w698 _ _ _ _ _ _]
          tunnel: "Sort out start and end positions" -> [_ _ _ _ _ w471 w478 w485 _ w504 _ w540 _ _ _ _ _ _ _ _ _ _ _]
          tunnel: "Check for Start NaNs" -> [w446 _ _ w461 w464 _ _ _ w494 _ _ w541 _ _ _ _ _ _ _ _ _ _ _]
          tunnel: [w442 w452 w456 w460 w465 w470 w477 w484 w495 w503 w517 w522 w598 w613 w626 w652 w701 w729 w734 w738 w750 w754 w758] -> w424
          tunnel: w423 -> [_ _ _ _ _ _ _ _ _ _ _ _ _ _ _ w658 _ _ _ _ _ _ _]
          frame "Move Traverse Only" {
            n162 = Unbundle By Name(w443) -> ("Specific Arguments"=w444:string)
            n163 = call <vilib>:"Trim Whitespace.vi"("string"=w444) -> ("trimmed string"=w438:string)  [unwired: 1 in]
            n164 = Equal?(x=w438, y="No Backlash") -> (x = y?=w441:bool)
            n165 = Empty String/Path?(string/path=w438) -> (empty?=w440:bool)
            n166 = Or(x=w440, y=w441) -> (x .or. y?=w439:bool)
            n167 = case shown="True" w439 {
              tunnel: w438 -> [w449 _]
              tunnel: [w448 ""] -> w437
              frame False {
                n168 = Format Into String(format string="\"%s\" is an Incorrect Specific Argument. It should either be left blank or say \"No Backlash\"\n", w449) -> (resulting string=w448:string)  [unwired: 2 in, 1 out]
              }
              frame True {
              }
            }
            n169 = Bundle By Name(cluster=w443, "Specific Arguments"=w438) -> (w442:T1)
          }
          frame "Set Tunnel Speed Only" {
          }
          frame "Set Source Only" {
          }
          frame "Set Measurement Conditions" {
          }
          frame "Single Measurement" {
            n170 = Build Array("Averaging:Time:(mins)" ("Label for value"), "Filename:HD:Users" ("Label for value")) -> (w466:string[])
          }
          frame "Vertical Profile" {
            n171 = Build Array("Number:Of:Points" ("Label for value"), "Averaging:Time:(mins)" ("Label for value"), "Filename:HD:Users" ("Label for value")) -> (w473:string[])
          }
          frame "Lateral Profile" {
            n172 = Build Array("Number:Of:Points" ("Label for value"), "Averaging:Time:(mins)" ("Label for value"), "Filename:HD:Users" ("Label for value")) -> (w480:string[])
          }
          frame "Longitudinal Profile" {
            n173 = Build Array("Number:Of:Points" ("Label for value"), "Averaging:Time:(mins)" ("Label for value"), "Filename:HD:Users" ("Label for value")) -> (w487:string[])
          }
          frame "Explore Volume" {
            n174 = Unbundle By Name(w495) -> ("Specific Arguments"=w493:string)
            n175 = Build Array("Averaging:Time:(mins)" ("Label for value"), "Filename:HD:Users" ("Label for value")) -> (w500:string[])
            n176 = Fract/Exp String To Number(string=w493) -> (number=w492:dbl)  [unwired: 4 out]
            n177 = Greater Than 0?(x=w492) -> (x > 0?=w491:bool)
            n178 = Format Into String(format string="\"%s\" is an Incorrect Specific Argument. Please enter the radius of the volume in mm.\n", w493) -> (resulting string=w497:string)  [unwired: 2 in, 1 out]
            n179 = Select(t="", s=w491, f=w497) -> (s? t:f=w496:string)
          }
          frame "Multi-Axis Profile" {
            n180 = Unbundle By Name(w503) -> ("Spacing"=w506:T2)
            n181 = case shown="\"Gauss\"" w506 {
              tunnel: ["" "You are not allowed to specify gaussian spacing for a Multi-Axis profile.\n" "You are not allowed to specify Log spacing for a Multi-Axis profile.\n" "\"N/A\" is not a valid point spacing.\n"] -> w505
              frame "Linear", Default {
              }
              frame "Gauss" {
              }
              frame "Log" {
              }
              frame "N/A" {
              }
            }
            n182 = Build Array("Number:Of:Points" ("Label for value"), "Averaging:Time:(mins)" ("Label for value"), "Filename:HD:Users" ("Label for value")) -> (w508:string[])
          }
          frame "Traverse 3D Volume" {
            n183 = Build Array("Averaging:Time:(mins)" ("Label for value"), "Filename:HD:Users" ("Label for value")) -> (w518:string[])
          }
          frame "Auto Calibrate" {
            n184 = Unbundle By Name(w521) -> ("Filename"=w525:path, "Specific Arguments"=w556:string)
            n185 = call "Get_array_values_fr_String.vi"("String Value"=w556) -> ("Numeric Array"=w552:dbl[], "String array"=w539:string[])
            n186 = global read "Trav_pos_global.vi" "Work in Tunnel Coordinates?"() -> (w535:T6)
            n187 = Index Array(array=w539, index=0 ("Index")) -> (element=w538:string)
            n188 = Build Array("Tunnel Speed", "Traverse Position", "Concentration") -> (w537:string[])
            n189 = Build Array("Averaging:Time:(mins)" ("Label for value")) -> (w543:string[])
            n190 = Array Size(array=w552) -> (size(s)=w551:i32)
            n191 = call "Current_Filepath.vi"("Filename in"=w525, "Data Type"="Calibrations") -> ("Filename Out"=w523:path)  [unwired: 1 out]
            n192 = Equal?(x=w535, y=Tunnel_Coordinates."Work in Model Coordinates" ("Work in Tunnel Coordinates?")) -> (x = y?=w529:bool)
            n193 = Search 1D Array(1D array=w537, element=w538) -> (index of element=w530:i32)  [unwired: 1 out]
            n194 = Equal?(x=2, y=w530) -> (x = y?=w532:bool)
            n195 = case shown="1" w530 {
              tunnel: [w586 w587] -> w542
              tunnel: w541 -> [w586 _]
              tunnel: w540 -> [_ w587]
              frame 0, Default {
              }
              frame 1 {
              }
            }
            n196 = Less?(x=w551, y=3) -> (x < y?=w547:bool)
            n197 = Equal To 0?(x=w530) -> (x = 0?=w548:bool)
            n198 = And(x=w529, y=w532) -> (x .and. y?=w531:bool)
            n199 = Greater Or Equal To 0?(x=w530) -> (x >= 0?=w528:bool)
            n200 = Compound Arithmetic op=AND(w547, w548) -> (w546:bool)
            n201 = case shown="True" w531 {
              tunnel: [w573 w578] -> w524
              tunnel: w521 -> [w573 w574]
              frame False {
              }
              frame True {
                n202 = global read "Extra_Commands_Global.vi" "Work in Tunnel Coordinates"() -> (w576:string)
                n203 = Unbundle By Name(w574) -> ("Extra Commands"=w575:string)
                n204 = call "Extra_Commands.vi"("String to Search"=w575, "Command"=w576) -> ("Command Found"=w577:bool)  [unwired: 1 in, 4 out]
                n205 = case shown="False" w577 {
                  tunnel: [w584 w585] -> w578
                  tunnel: w576 -> [w583 _]
                  tunnel: w575 -> [w582 _]
                  tunnel: w574 -> [w580 w585]
                  frame False {
                    n206 = Concatenate Strings(w583, "  " ("string"), w582) -> (w581:string)
                    n207 = Bundle By Name(cluster=w580, "Extra Commands"=w581) -> (w584:T1)
                  }
                  frame True {
                  }
                }
              }
            }
            n208 = Select(t="You need to enter the desired tunnel speeds in the \"Specfic Arguments\" Box   eg.  Tunnel Speed;1;2;3;4\n", s=w546, f="") -> (s? t:f=w544:string)
            n209 = call "Does_file_exist_(simple).vi"("Pathname"=w523) -> ("exists?"=w562:bool)
            n210 = case shown="False" w528 {
              tunnel: w537 -> [w564 _]
              tunnel: [w563 ""] -> w527
              frame False {
                n211 = for {
                  shift-right: [w569] -> w566
                  shift-left: "Incorrect Specific Argument. The options are: " -> [w570]
                  tunnel: w564 -> [w571] mode=indexing
                  w568 = "  " ("Substring")
                  n212 = Concatenate Strings(w570, w568, w571, w568) -> (w569:string)
                }
                n213 = Concatenate Strings(w566, "\r\n") -> (w563:string)
              }
              frame True {
              }
            }
            n214 = Select(t="", s=w562, f="The calibration file cannot be found.\n") -> (s? t:f=w558:string)
            n215 = Bundle By Name(cluster=w524, "Filename"=w523) -> (w522:T1)
            n216 = Concatenate Strings(w558, w544, w527) -> (w557:string)
          }
          frame "Meas Fast FID Bkgnd" {
            n217 = Unbundle By Name(w598) -> ("Specific Arguments"=w593:string)
            n218 = call "Get_array_values_fr_String.vi"("String Value"=w593) -> ("String array"=w592:string[])  [unwired: 1 out]
            n219 = Index Array(array=w592, index=0) -> (element=w590:string)
            n220 = Empty String/Path?(string/path=w590) -> (empty?=w596:bool)
            n221 = Build Array("Averaging:Time:(mins)" ("Label for value")) -> (w600:string[])
            n222 = Equal?(x=w590, y="Use Source Divertor Valve") -> (x = y?=w589:bool)
            n223 = Or(x=w596, y=w589) -> (x .or. y?=w595:bool)
            n224 = case shown="False" w595 {
              tunnel: ["Specific Argument should either be blank or\nUse Source Divertor Valve ; (wait time in seconds optional)" ""] -> w594
              frame False {
              }
              frame True {
              }
            }
          }
          frame "Check Beam Power" {
            n225 = Unbundle By Name(w605) -> ("Extra Commands"=w607:string, "Start X"=w612:dbl, "Start Y"=w610:dbl, "Start Z"=w611:dbl)
            n226 = global read "Extra_Commands_Global.vi" "Skip Traverse Position Demand"() -> (w608:string)
            n227 = call "Extra_Commands.vi"("String to Search"=w607, "Command"=w608) -> ("Command Found"=w606:bool)  [unwired: 1 in, 4 out]
            n228 = case shown="False" w606 {
              tunnel: w612 -> [w624 _]
              tunnel: w611 -> [w623 _]
              tunnel: w610 -> [w622 _]
              tunnel: "" -> [w619 w625]
              tunnel: [w618 w625] -> w604
              frame False {
                n229 = Build Array(w624, w622, w623) -> (w621:dbl[])
                n230 = Not A Number/Path/Refnum?(number/path/refnum=w621) -> (NaN/Path/Refnum?=w620:bool[])
                n231 = Or Array Elements(Boolean array=w620) -> (logical OR=w617:bool)
                n232 = Select(t="The start position is where the datum velocity measurement will be made. This should not contain NaNs.\n" ("f"), s=w617, f=w619) -> (s? t:f=w618:string)
              }
              frame True {
              }
            }
            n233 = Bundle By Name(cluster=w605, "Comments"="Start Position is the location of Datum Velocity Measurement") -> (w613:T1)
          }
          frame "Scanning Valve Measurement" {
            w639 = ext -0.5  # lo
            w640 = ext 47.5  # hi
            n234 = Unbundle By Name(w626) -> ("Specific Arguments"=w636:string)
            n235 = call "Get_array_values_fr_String.vi"("String Value"=w636) -> ("Numeric Array"=w635:dbl[], "String array"=w631:string[])
            n236 = Build Array("Averaging:Time:(mins)" ("Label for value"), "Filename:HD:Users" ("Label for value")) -> (w643:string[])
            n237 = Index Array(array=w631, index=0) -> (element=w630:string)
            n238 = Empty String/Path?(string/path=w630) -> (empty?=w628:bool)
            n239 = Index Array(array=w635, index=0) -> (element=w633:dbl)
            n240 = In Range and Coerce(upper limit=w640, x=w633, lower limit=w639) -> (In Range?=w629:bool)  [unwired: 1 out]
            n241 = Compound Arithmetic op=AND(invert w628, w629) -> (w627:bool)
            n242 = Select(t="", s=w627, f="Enter the scanning valve port number between 0 and 47 in the specific arguments box.\n") -> (s? t:f=w638:string)
          }
          frame "Set ADAM Ch" {
            n243 = Unbundle By Name(w653) -> ("Specific Arguments"=w664:string, "Extra Commands"=w646:string)
            n244 = while {
              shift-right: [w691] -> w660
              shift-left: _ -> [w684]
              shift-right: [w690] -> _
              shift-left: _ -> [w689]
              tunnel: w658 -> [w690]
              stop <- TRUE stop-if-true
              n245 = Array Size(array=w684) -> (size(s)=w688:i32)
              n246 = Less?(x=w690, y=w689) -> (x < y?=w686:bool)
              n247 = Equal To 0?(x=w688) -> (x = 0?=w687:bool)
              n248 = Or(x=w687, y=w686) -> (x .or. y?=w685:bool)
              n249 = case shown="True" w685 {
                tunnel: [w692 w693] -> w691
                tunnel: w684 -> [w692 _]
                frame False {
                }
                frame True {
                  n250 = call "Get_ADAM_Ch_names_client.vi"("Channel names set"=Channel_names."Active + Off") -> ("Ch names"=w693:string[])
                }
              }
            }
            n251 = call "Get_array_values_fr_String.vi"("String Value"=w664) -> ("String array"=w651:string[])  [unwired: 1 out]
            n252 = Index Array(array=w651, index=0) -> (element=w659:string)
            n253 = Empty String/Path?(string/path=w646) -> (empty?=w649:bool)
            n254 = Search 1D Array(1D array=w660, element=w659) -> (index of element=w662:i32)  [unwired: 1 out]
            n255 = Greater Or Equal To 0?(x=w662) -> (x >= 0?=w661:bool)
            n256 = Select(t="You have not specified a Value to Set the ADAM channel to.\nPlease give a value in the Extra Commands string", s=w649, f="") -> (s? t:f=w647:string)
            n257 = case shown="True" w661 {
              tunnel: w660 -> [w678 _]
              tunnel: w659 -> [w676 w679]
              tunnel: w658 -> [w674 _]
              tunnel: [w672 FALSE ("Cancel")] -> w657
              tunnel: w653 -> [w668 w681]
              tunnel: [w667 w680] -> w652
              tunnel: w646 -> [_ _]
              frame False {
                n258 = Build Array(w676) -> (w675:string[])
                n259 = Format Into String(format string="Please Select the ADAM Channel that you want to set in row %d", w674) -> (resulting string=w673:string)  [unwired: 2 in, 1 out]
                n260 = call "Select_Strings.vi"("Available Ch names"=w678, "Message"=w673, "Selector mode"=T7."One", "Desired Ch names (in)"=w675) -> ("Cancel"=w672:bool, "Selected Channel Names"=w670:string[])  [unwired: 3 out]
                n261 = Index Array(array=w670, index=0) -> (element=w666:string)
                n262 = Bundle By Name(cluster=w668, "Specific Arguments"=w666) -> (w667:T1)
              }
              frame True {
                n263 = Bundle By Name(cluster=w681, "Specific Arguments"=w679) -> (w680:T1)
              }
            }
            n264 = Select(t="Close Front Panel", s=w657, f=w655) -> (s? t:f=w656:string)
          }
          frame "Run VI Named:" {
            w706 = "Run_VI_Named_specific.vi"
            n265 = Unbundle By Name(w701) -> ("Specific Arguments"=w709:string)
            n266 = global read "Constants_global.vi" "Run VI Folder"() -> (w707:path)
            n267 = Match Pattern(string=w709, regular expression=";") -> (before substring=w710:string)  [unwired: 4 out]
            n268 = call <vilib>:"Trim Whitespace.vi"("string"=w710) -> ("trimmed string"=w702:string)  [unwired: 1 in]
            n269 = call "Run_VI_Named_specific.vi"("Run VI Named String"=w702, "Multi Run Row"=w701) -> ("Checks"=w696:string[], "Error String"=w695:string, "Check for start NaNs?"=w700:bool)  [unwired: 7 out]
            n270 = Select(t="Check for Start NaNs" ("Label for value"), s=w700, f=w698) -> (s? t:f=w697:string)
            n271 = Build Path(base path=w707, name or relative path=w702) -> (appended path=w713:path)
            n272 = Not Equal?(x=w702, y=w706) -> (x != y?=w705:bool)
            n273 = call "Does_file_exist_(simple).vi"("Pathname"=w713) -> ("exists?"=w704:bool)
            n274 = And(x=w704, y=w705) -> (x .and. y?=w703:bool)
            n275 = case shown="False" w703 {
              tunnel: [w720 ""] -> w708
              tunnel: w707 -> [w716 _]
              tunnel: w706 -> [w714 _]
              frame False {
                w718 = "\r\n"
                n276 = Build Array(w714) -> (w715:string[])
                n277 = call "List_files_in_order_of_age.vi"("Files to Hide"=w715, "Folder"=w716) -> ("file names"=w717:string[])
                n278 = for {
                  shift-right: [w724] -> w721
                  shift-left: "Cannot find the VI to run. Specific Argument options are:" -> [w725]
                  tunnel: w717 -> [w726] mode=indexing
                  w723 = "  " ("Substring")
                  n279 = Concatenate Strings(w725, w723, w726, w723) -> (w724:string)
                }
                n280 = Concatenate Strings(w721, w718, "Please place one of these strings in the \"Specific Argument\" field.", w718) -> (w720:string)
              }
              frame True {
              }
            }
            n281 = Concatenate Strings(w695, w708) -> (w712:string)
          }
          frame "Wait (minutes)" {
            n282 = Unbundle By Name(w729) -> ("Specific Arguments"=w730:string)
            n283 = call "Wait_Case_Arg.vi"("Specific Argument"=w730) -> ("Error Comments"=w731:string)  [unwired: 1 in, 4 out]
          }
          frame "Send Message" {
          }
          frame "Synchronize With:" {
            n284 = local read "Current Sync Number"() -> (w739:i32)
            n285 = call "Synchronize_Prog_Arg.vi"("Execution Row"=w738) -> ("Error Comments"=w741:string, "Sync No"=w747:i32)  [unwired: 3 out]
            n286 = Equal?(x=w747, y=w739) -> (x = y?=w746:bool)
            n287 = Format Into String(format string="This should be Synchroisation number %d.\n" ("Format String"), w739) -> (resulting string=w744:string)  [unwired: 2 in, 1 out]
            n288 = Select(t="", s=w746, f=w744) -> (s? t:f=w742:string)
            n289 = Concatenate Strings(w742, w741) -> (w740:string)
          }
          frame "Fall Back to this Row" {
          }
          frame "Turn Off Row Repeating" {
          }
          frame "Blank Row" {
            n290 = Unbundle By Name(w760) -> ("Comments"=w766:string)
            n291 = Match Pattern(string=w766, regular expression="(No Match Info)") -> (before substring=w759:string, after substring=w763:string)  [unwired: 3 out]
            n292 = Empty String/Path?(string/path=w763) -> (empty?=w764:bool)
            n293 = Bundle By Name(cluster=w760, "Comments"=w759) -> (w758:T1)
            n294 = Select(t=w763, s=w764, f="The Row Type Selector \"%s\" was not matched. Please select the desired type.\n") -> (s? t:f=w762:string)
          }
        }
        "Checks" <- w431
        n295 = Concatenate Strings(w434, w435) -> (w433:string)
      }
      frame "Sort out start and end positions" {
        n296 = Unbundle By Name(w774) -> ("Start X"=w786:dbl, "Start Y"=w785:dbl, "Start Z"=w784:dbl, "End X"=w783:dbl, "End Y"=w782:dbl, "End Z"=w781:dbl, "Extra Commands"=w770:string)
        n297 = call "Which_Trav_Setup.vi"("Extra Command String"=w770) -> ("Traverse Setups"=w768:string[])
        n298 = Build Array(w786, w785, w784) -> (w777:dbl[])
        n299 = Build Array(w783, w782, w781) -> (w776:dbl[])
        n300 = Index Array(array=w768) -> (element=w769:string)  [unwired: 1 in]
        n301 = call "Rig_Pict_Display_Pref.vi"("Traverse Name"=w769) -> ("Which Axis is vertical?"=w780:enum16{"X Axis", "Y Axis", "Z Axis"})  [unwired: 7 out]
        n302 = case shown="\"Multi-Axis Profile\", Default" w775 {
          tunnel: [w826 FALSE w842 w855 FALSE] -> w789
          tunnel: [w825 FALSE w841 w854 FALSE] -> w788
          tunnel: [w824 FALSE w840 w853 FALSE] -> w787
          tunnel: w780 -> [w823 _ w839 w852 _]
          frame "Vertical Profile" {
            n303 = case shown="\"Z Axis\"" w823 {
              tunnel: [FALSE TRUE TRUE] -> w826
              tunnel: [TRUE FALSE TRUE] -> w825
              tunnel: [TRUE TRUE FALSE] -> w824
              frame "X Axis" {
              }
              frame "Y Axis" {
              }
              frame "Z Axis" {
              }
            }
          }
          frame "Auto Calibrate" {
          }
          frame "Lateral Profile" {
            n304 = case shown="\"Y Axis\"" w839 {
              tunnel: [TRUE TRUE TRUE] -> w842
              tunnel: [TRUE TRUE FALSE] -> w841
              tunnel: [FALSE FALSE TRUE] -> w840
              frame "X Axis" {
              }
              frame "Y Axis" {
              }
              frame "Z Axis" {
              }
            }
          }
          frame "Longitudinal Profile" {
            n305 = case shown="\"Y Axis\"" w852 {
              tunnel: [FALSE FALSE FALSE] -> w855
              tunnel: [TRUE TRUE TRUE] -> w854
              tunnel: [TRUE TRUE TRUE] -> w853
              frame "X Axis" {
              }
              frame "Y Axis" {
              }
              frame "Z Axis" {
              }
            }
          }
          frame "Multi-Axis Profile", Default {
          }
        }
        n306 = Build Array(w789, w788, w787) -> (w778:bool[])
        "Fixed Axis" <- w778
        n307 = for {
          tunnel: w778 -> [w796] mode=indexing
          tunnel: w777 -> [w795] mode=indexing
          tunnel: w776 -> [w794] mode=indexing
          shift-right: [w791] -> w773
          shift-left: w774 -> [w792]
          i -> [w793]
          n308 = case shown="True" w796 {
            tunnel: w795 -> [_ w802]
            tunnel: w794 -> [_ w801]
            tunnel: w793 -> [_ w800]
            tunnel: w792 -> [w797 w799]
            tunnel: [w797 w798] -> w791
            frame False {
            }
            frame True {
              n309 = Not A Number/Path/Refnum?(number/path/refnum=w802) -> (NaN/Path/Refnum?=w803:bool)
              n310 = Not A Number/Path/Refnum?(number/path/refnum=w801) -> (NaN/Path/Refnum?=w805:bool)
              n311 = Exclusive Or(1:w805, 2:w803) -> (0:w804:bool)
              n312 = case shown="True" w804 {
                tunnel: w803 -> [_ w813]
                tunnel: w802 -> [_ w812]
                tunnel: w801 -> [_ w811]
                tunnel: w800 -> [_ w810]
                tunnel: w799 -> [w806 w809]
                tunnel: [w806 w808] -> w798
                frame False {
                }
                frame True {
                  n313 = Select(t=w811, s=w813, f=w812) -> (s? t:f=w807:dbl)
                  n314 = case shown="2" w810 {
                    tunnel: w809 -> [w816 w819 w822]
                    tunnel: [w815 w818 w821] -> w808
                    tunnel: w807 -> [w814 w817 w820]
                    frame 0, Default {
                      n315 = Bundle By Name(cluster=w816, "Start X"=w814, "End X"=w814) -> (w815:T1)
                    }
                    frame 1 {
                      n316 = Bundle By Name(cluster=w819, "Start Y"=w817, "End Y"=w817) -> (w818:T1)
                    }
                    frame 2 {
                      n317 = Bundle By Name(cluster=w822, "Start Z"=w820, "End Z"=w820) -> (w821:T1)
                    }
                  }
                }
              }
            }
          }
        }
      }
      frame "Check for position NaNs" {
        n318 = global read "Extra_Commands_Global.vi" "Skip Traverse Position Demand"() -> (w871:string)
        n319 = Unbundle By Name(w874) -> ("Extra Commands"=w870:string, "Start X"=w883:dbl, "Start Y"=w881:dbl, "Start Z"=w882:dbl, "End X"=w880:dbl, "End Y"=w879:dbl, "End Z"=w878:dbl)
        n320 = call "Extra_Commands.vi"("String to Search"=w870, "Command"=w871) -> ("Command Found"=w868:bool)  [unwired: 1 in, 4 out]
        n321 = case shown="False" w868 {
          tunnel: w883 -> [w898 _]
          tunnel: w882 -> [w897 _]
          tunnel: w881 -> [w896 _]
          tunnel: w880 -> [w895 _]
          tunnel: w879 -> [w894 _]
          tunnel: w878 -> [w893 _]
          tunnel: [w889 w899] -> w877
          tunnel: [w888 TRUE] -> w876
          tunnel: "" -> [w887 w899]
          frame False {
            n322 = Build Array(w898, w896, w897, w895, w894, w893) -> (w892:dbl[])
            n323 = Not A Number/Path/Refnum?(number/path/refnum=w892) -> (NaN/Path/Refnum?=w891:bool[])
            n324 = Or Array Elements(Boolean array=w891) -> (logical OR=w888:bool)
            n325 = Select(t="Some of the Start and End positions are NaN.\n" ("f"), s=w888, f=w887) -> (s? t:f=w889:string)
          }
          frame True {
          }
        }
        n326 = case shown="\"Set Tunnel Speed Only\", Default" w872 {
          tunnel: w876 -> [_ w905]
          tunnel: ["Check source details" ("t") w904] -> w875
          frame "Multi-Axis Profile" {
          }
          frame "Set Tunnel Speed Only", Default {
            n327 = Select(t="Check source details", s=w905, f="Check profile rows") -> (s? t:f=w904:string)
          }
        }
        n328 = Concatenate Strings(w885, w877) -> (w884:string)
      }
      frame "Check for Start NaNs" {
        n329 = Unbundle By Name(w911) -> ("Extra Commands"=w907:string, "Start X"=w916:dbl, "Start Y"=w914:dbl, "Start Z"=w915:dbl)
        n330 = global read "Extra_Commands_Global.vi" "Skip Traverse Position Demand"() -> (w908:string)
        n331 = call "Extra_Commands.vi"("String to Search"=w907, "Command"=w908) -> ("Command Found"=w906:bool)  [unwired: 1 in, 4 out]
        n332 = case shown="True" w906 {
          tunnel: w916 -> [w928 _]
          tunnel: w915 -> [w927 _]
          tunnel: w914 -> [w926 _]
          tunnel: "" -> [w923 w929]
          tunnel: [w921 w929] -> w912
          frame False {
            n333 = Build Array(w928, w926, w927) -> (w925:dbl[])
            n334 = Not A Number/Path/Refnum?(number/path/refnum=w925) -> (NaN/Path/Refnum?=w924:bool[])
            n335 = Or Array Elements(Boolean array=w924) -> (logical OR=w920:bool)
            n336 = Select(t="Some of the Start coordinates are NaN.\n" ("f"), s=w920, f=w923) -> (s? t:f=w921:string)
          }
          frame True {
          }
        }
        n337 = Concatenate Strings(w918, w912) -> (w917:string)
      }
      frame "Check profile rows" {
        n338 = call "Create_Pos_array.vi"("Traverse line"=w939) -> ("Traverse line Out"=w938:T1, "Error Messages"=w937:string)  [unwired: 7 out]
        n339 = Unbundle By Name(w939) -> ("Start X"=w961:dbl, "Start Y"=w960:dbl, "Start Z"=w959:dbl, "End X"=w958:dbl, "End Y"=w957:dbl, "End Z"=w956:dbl, "Specific Arguments"=w950:string, "Spacing"=w945:T2, "No. of pts."=w944:i32)
        n340 = local read "Fixed Axis"() -> (w943:bool[])
        n341 = Build Array(w961, w960, w959) -> (w941:dbl[])
        n342 = Build Array(w958, w957, w956) -> (w942:dbl[])
        n343 = case shown="\"Linear\"" w945 {
          tunnel: w950 -> [_ _ _ _ w996]
          tunnel: ["" w969 "\"N/A\" is not a valid point spacing.\n" "" w991] -> w949
          tunnel: w944 -> [_ _ _ _ w995]
          tunnel: w943 -> [_ w967 _ _ _]
          tunnel: w942 -> [_ w974 _ _ _]
          tunnel: w941 -> [_ w973 _ _ _]
          frame "Linear" {
          }
          frame "Log" {
            n344 = for {
              tunnel: w974 -> [w978] mode=indexing
              tunnel: w973 -> [w977] mode=indexing
              tunnel: [w976] -> w972 mode=indexing
              tunnel: w967 -> [w975] mode=indexing
              n345 = case shown="False" w975 {
                tunnel: w978 -> [w984 _]
                tunnel: w977 -> [w983 _]
                tunnel: [w979 FALSE] -> w976
                frame False {
                  w982 = 0.001 ("y")
                  n346 = Less?(x=w984, y=w982) -> (x < y?=w980:bool)
                  n347 = Less?(x=w983, y=w982) -> (x < y?=w981:bool)
                  n348 = Or(x=w980, y=w981) -> (x .or. y?=w979:bool)
                }
                frame True {
                }
              }
            }
            n349 = Or Array Elements(Boolean array=w972) -> (logical OR=w971:bool)
            n350 = Select(t="For log spacing, Start & End positions must be greater than 0.0001.", s=w971, f="") -> (s? t:f=w969:string)
          }
          frame "N/A" {
          }
          frame "Gauss" {
          }
          frame "Specified" {
            n351 = call "Get_array_values_fr_String.vi"("String Value"=w996) -> ("Numeric Array"=w990:dbl[])  [unwired: 1 out]
            n352 = Array Size(array=w990) -> (size(s)=w989:i32)
            n353 = Decrement(x=w989) -> (x-1=w988:i32)
            n354 = Equal?(x=w988, y=w995) -> (x = y?=w994:bool)
            n355 = Select(t="", s=w994, f="The No of points and No of Arguments do not match.\n") -> (s? t:f=w991:string)
          }
        }
        n356 = for {
          tunnel: w943 -> [w1002] mode=indexing
          tunnel: w941 -> [w1001] mode=indexing
          tunnel: w942 -> [w1000] mode=indexing
          tunnel: [w999] -> w955 mode=indexing
          shift-right: [w997] -> w934
          shift-left: bool[] [] -> [w998]
          n357 = case shown="False" w1002 {
            tunnel: w1001 -> [w1006 w1012]
            tunnel: w1000 -> [w1007 w1011]
            tunnel: [TRUE w1010] -> w999
            tunnel: w998 -> [w1004 w1009]
            tunnel: [w1003 w1009] -> w997
            frame False {
              n358 = Not Equal?(x=w1006, y=w1007) -> (x != y?=w1005:bool)
              n359 = Build Array (concatenate)(w1004, w1005) -> (w1003:bool[])
            }
            frame True {
              n360 = Equal?(x=w1012, y=w1011) -> (x = y?=w1010:bool)
            }
          }
        }
        n361 = Array Size(array=w934) -> (size(s)=w933:i32)
        n362 = And Array Elements(Boolean array=w955) -> (logical AND=w954:bool)
        n363 = Or Array Elements(Boolean array=w934) -> (logical OR=w931:bool)
        n364 = Not Equal To 0?(x=w933) -> (x != 0?=w932:bool)
        n365 = And(x=w931, y=w932) -> (x .and. y?=w930:bool)
        n366 = Select(t="", s=w954, f="This profile moves more than one axis.\n") -> (s? t:f=w951:string)
        n367 = Select(t="", s=w930, f="The start and end points are the same for this profile.\n") -> (s? t:f=w947:string)
        n368 = Concatenate Strings(w937, w947, w951, w949) -> (w964:string)
        n369 = Concatenate Strings(w963, w964) -> (w962:string)
      }
      frame "Check source details" {
        n370 = Unbundle By Name(w1024) -> ("Emission Rate (l/min)"=w1026:dbl, "Density Ratio"=w1016:string)  [unwired: 1 out]
        n371 = Empty String/Path?(string/path=w1016) -> (empty?=w1017:bool)
        n372 = Equal?(x=w1016, y="---------" ("f")) -> (x = y?=w1015:bool)
        n373 = Or(x=w1017, y=w1015) -> (x .or. y?=w1014:bool)
        n374 = Greater Than 0?(x=w1026) -> (x > 0?=w1021:bool)
        n375 = And(x=w1021, y=w1014) -> (x .and. y?=w1025:bool)
        n376 = case shown="False" w1025 {
          tunnel: w1024 -> [w1029 w1032]
          tunnel: [w1029 w1030] -> w1023
          frame False {
          }
          frame True {
            (unwired) "The Density Ratio Box should contain either:\nCarrier 1 Only\nCarrier 2 Only\nor the relative density ratio of the mixed gas with respect to air" ("f")
            n377 = Bundle By Name(cluster=w1032, "Density Ratio"="Carrier 1 Only") -> (w1030:T1)
          }
        }
        n378 = Select(t="Check source detail 2", s=w1021, f="check entered filename etc") -> (s? t:f=w1019:string)
      }
      frame "Check source detail 2" {
        n379 = Unbundle By Name(w1056) -> ("Trace Gas Concentration (%)"=w1057:dbl, "Density Ratio"=w1058:string)
        n380 = To Upper Case(1:w1058) -> (0:w1041:string)
        n381 = To Upper Case(1:"Carrier 1 Only") -> (0:w1043:string)
        n382 = To Upper Case(1:"Carrier 2 Only") -> (0:w1042:string)
        n383 = In Range and Coerce(upper limit=ext 3.01 ("hi"), x=w1057, lower limit=ext 0.0 ("lo")) -> (In Range?=w1038:bool)  [unwired: 1 out]
        n384 = Equal?(x=w1041, y=w1043) -> (x = y?=w1048:bool)
        n385 = Equal?(x=w1041, y=w1042) -> (x = y?=w1047:bool)
        n386 = Fract/Exp String To Number(string=w1041) -> (number=w1049:dbl)  [unwired: 4 out]
        n387 = In Range and Coerce(upper limit=ext 10.0 ("hi"), x=w1049, lower limit=ext 0.05 ("lo")) -> (In Range?=w1046:bool)  [unwired: 1 out]
        n388 = Compound Arithmetic op=OR(w1048, w1047, w1046) -> (w1033:bool)
        n389 = Select(t="", s=w1038, f="The Trace Gas Concentration must be within the range of 0 to 3%.\n") -> (s? t:f=w1034:string)
        n390 = Select(t="", s=w1033, f="The Density Ratio Box should contain either:\nCarrier 1 Only\nCarrier 2 Only\nor the relative density ratio of the mixed gas with respect to air") -> (s? t:f=w1035:string)
        n391 = Concatenate Strings(w1034, w1035) -> (w1059:string)
        n392 = Concatenate Strings(w1061, w1059) -> (w1060:string)
      }
      frame "check entered filename etc" {
        n393 = local read "Checks"() -> (w1074:string[])
        n394 = for {
          tunnel: w1074 -> [w1081] mode=indexing
          tunnel: [w1086] -> w1075 mode=indexing
          tunnel: w1071 -> [w1085]
          shift-right: [w1083] -> w1065
          shift-left: w1066 -> [w1084]
          tunnel: [w1082] -> w1064 mode=indexing
          n395 = case shown="\"Number:Of:Points\"" w1081 {
            tunnel: w1084 -> [w1088 w1096 w1118 w1133]
            tunnel: [w1089 w1099 w1124 w1129] -> w1086
            tunnel: w1085 -> [_ _ w1127 _]
            tunnel: [w1088 w1096 w1116 w1133] -> w1083
            tunnel: [TRUE ("cancelled") TRUE ("cancelled") w1111 TRUE ("cancelled")] -> w1082
            tunnel: w1081 -> [_ _ _ w1131]
            frame "Number:Of:Points" {
              n396 = Unbundle By Name(w1088) -> ("No. of pts."=w1091:i32)
              n397 = Greater?(x=w1091, y=0) -> (0:w1093:bool)
              n398 = Select(t="", s=w1093, f="For a profile the number of points should be more than 0.\n" ("Format String")) -> (s? t:f=w1089:string)
            }
            frame "Averaging:Time:(mins)" {
              n399 = Unbundle By Name(w1096) -> ("Averaging time (min)"=w1098:dbl)
              n400 = Greater Than 0?(x=w1098) -> (x > 0?=w1097:bool)
              n401 = Select(t="", s=w1097, f="The averaging time should be greater than zero.\n" ("Format String")) -> (s? t:f=w1099:string)
            }
            frame "Filename:HD:Users" {
              w1125 = FALSE  # Show Error handler
              n402 = Unbundle By Name(w1118) -> ("Filename"=w1102:path, "Row No"=w1113:i32, "Row Type Selector"=w1109:T3)
              n403 = call "Row_type_selector_string.vi"("Mode"=w1109) -> ("Output string"=w1108:string)
              n404 = call "Current_Filepath.vi"("Filename in"=w1102, "Data Type"="Results") -> ("Filename Out"=w1103:path)  [unwired: 1 out]
              n405 = Path To String(path=w1103) -> (string=w1122:string)
              n406 = Not A Number/Path/Refnum?(number/path/refnum=w1103) -> (NaN/Path/Refnum?=w1106:bool)
              n407 = Equal?(x=Multi_run_mode."Run VI Named:" ("Mode"), y=w1127) -> (x = y?=w1126:bool)
              n408 = Match Pattern(string=w1122, regular expression="-------" ("f")) -> (match substring=w1121:string)  [unwired: 4 out]
              n409 = Empty String/Path?(string/path=w1121) -> (empty?=w1107:bool)
              n410 = Format Into String(format string=" For Row  %d %s." ("Comment"), w1113, w1108) -> (resulting string=w1112:string)  [unwired: 2 in, 1 out]
              n411 = Compound Arithmetic op=AND(w1107, invert w1106) -> (w1105:bool)
              n412 = Select(t=w1103, s=w1105, f=path "") -> (s? t:f=w1120:path)
              n413 = call "Results_filename_checker.vi"("Filelength"=45, "Warn if Already Exists"=w1126, "Comment"=w1112, "Show Error handler"=w1125, "Results file"=w1120) -> ("Error String"=w1124:string, "cancelled"=w1115:bool, "Results file output"=w1117:path)  [unwired: 1 out]
              n414 = Bundle By Name(cluster=w1118, "Filename"=w1117) -> (w1116:T1)
              n415 = Not(x=w1115) -> (.not. x?=w1111:bool)
            }
            frame "No Match", Default {
              n416 = Concatenate Strings(w1131, " Has not been programmed.\n" ("string")) -> (w1129:string)
            }
          }
        }
        n417 = local read "Editted Row"() -> (w1068:bool)
        n418 = And Array Elements(Boolean array=w1064) -> (logical AND=w1063:bool)
        n419 = Concatenate Strings(w1075) -> (w1073:string)
        n420 = Concatenate Strings(w1072, w1073) -> (w1067:string)
        n421 = Empty String/Path?(string/path=w1067) -> (empty?=w1070:bool)
        n422 = case shown="False" w1070 {
          tunnel: ["Open Front Panel" w1079] -> w1069
          tunnel: w1068 -> [_ w1080]
          frame False {
          }
          frame True {
            n423 = Select(t="Close Front Panel", s=w1080, f="End") -> (s? t:f=w1079:string)
          }
        }
      }
      frame "Open Front Panel" {
        w1138 = TRUE  # Front Panel Window:Open
        n424 = Current VI's Path() -> (path=w1139:path)
        n425 = call "Open_Close_Front_Panel.ph.vi"("Front Panel Window:Open"=w1138, "VI path"=w1139) -> ()  [unwired: 2 out]
        n426 = local write "Editted Row"(TRUE ("Editted Row")) -> ()
        n427 = local write "Execution Row"(w1135) -> ()
      }
      frame "What to do next?" {
        w1149 = ""
        w1147 = "[\r\n]"
        n428 = local read "Execution Row"() -> (w1145:T1)
        n429 = Unbundle By Name(w1145) -> ("Row Type Selector"=w1161:T3, "Specific Arguments"=w1156:string, "Extra Commands"=w1154:string, "Density Ratio"=w1148:string)
        n430 = Wait Until Next ms Multiple(millisecond multiple=u32 100) -> ()  [unwired: 1 out]
        n431 = Not Equal?(x=Multi_run_mode."Blank Row" ("Mode"), y=w1161) -> (x != y?=w1157:bool)
        n432 = call "Replace_Character.vi"("Replace with"=w1149, "Input String"=w1156, "Search For"=w1147) -> ("Output string"=w1155:string)  [unwired: 1 out]
        n433 = call "Replace_Character.vi"("Replace with"=w1149, "Input String"=w1154, "Search For"=w1147) -> ("Output string"=w1153:string)  [unwired: 1 out]
        n434 = call "Replace_Character.vi"("Replace with"=w1149, "Input String"=w1148, "Search For"=w1147) -> ("Output string"=w1146:string)  [unwired: 1 out]
        n435 = Compound Arithmetic op=OR("Edit in Excel", "OK") -> (w1158:bool)
        n436 = Bundle By Name(cluster=w1145, "Specific Arguments"=w1155, "Extra Commands"=w1153, "Density Ratio"=w1146) -> (w1143:T1)
        n437 = Compound Arithmetic op=AND(w1158, w1157) -> (w1151:bool)
        n438 = Not Equal?(x=w1143, y=w1145) -> (x != y?=w1144:bool)
        n439 = Not(x="Edit in Excel") -> (.not. x?=w1142:bool)
        n440 = case shown="True" w1144 {
          tunnel: w1143 -> [_ w1165]
          frame False {
          }
          frame True {
            n441 = local write "Execution Row"(w1165) -> ()
          }
        }
        n442 = case shown="True" w1142 {
          tunnel: ["Close Front Panel" w1170] -> w1150
          tunnel: w1151 -> [_ w1169]
          frame False {
          }
          frame True {
            n443 = Select(t="Clean Up Row", s=w1169, f="What to do next?") -> (s? t:f=w1170:string)
          }
        }
        "Error Comments" <- w1152
      }
      frame "Clean Up Row" {
        n444 = call "Traverse_Control_Ch_Names.vi"("Mode"=T4."All Channel Names") -> ("Channel names"=w1179:string[])  [unwired: 1 in]
        n445 = call "Trav_Cluster_to_Row.vi"("Traverse line in"=w1174, "Row Number"=w1175, "Channel names"=w1179) -> ("Traverse line Out"=w1177:T1)  [unwired: 4 out]
      }
      frame "Close Front Panel" {
        w1183 = FALSE  # Front Panel Window:Open
        n446 = Current VI's Path() -> (path=w1184:path)
        n447 = call "Open_Close_Front_Panel.ph.vi"("Front Panel Window:Open"=w1183, "VI path"=w1184) -> ()  [unwired: 2 out]
      }
      frame "End" {
        n448 = local read "Editted Row"() -> (w1192:bool)
        n449 = case shown="True" w1192 {
          tunnel: w1191 -> [w1195 w1198]
          tunnel: [w1195 w1197] -> w1189
          tunnel: w1190 -> [_ w1196]
          frame False {
          }
          frame True {
            n450 = call "Traverse_Control_Ch_Names.vi"("Mode"=T4."All Channel Names") -> ("Channel names"=w1199:string[])  [unwired: 1 in]
            n451 = call "Trav_Cluster_to_Row.vi"("Traverse line in"=w1198, "Row Number"=w1196, "Channel names"=w1199) -> ("Traverse line Out"=w1197:T1)  [unwired: 4 out]
          }
        }
        n452 = local write "Error Comments"(w1193) -> ()
      }
    }
    "Traverse line Out" <- w8
  }
  "Execution Row Out" <- w2
  "Continue?" <- w1
